vi "LoadMotorData.vi"(11 "Refnum in":T1) -> (3 "Refnum out":T1)   [LabVIEW 2014]
uses:
  <vilib>/Utility/config.llb/Config Data RefNum.ctl
  Variables/Physical data.vi
  <vilib>/Utility/config.llb/Read Key (Double).vi
  <vilib>/Utility/config.llb/Write Key (Double).vi
  <vilib>/Utility/config.llb/NI_LVConfig.lvlib
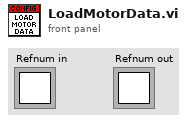
[diagram p1: front panel]
types:
  T1 = typedef "NI_LVConfig.lvlib/Config Data RefNum.ctl" = refnum<k1>
  T2 = cluster{"Free Current":dbl, "Stall Current":dbl, "Stall Torque":dbl, "Free Speed":dbl, "Gear Ratio":dbl, "Efficiency":dbl, "Moment":dbl}
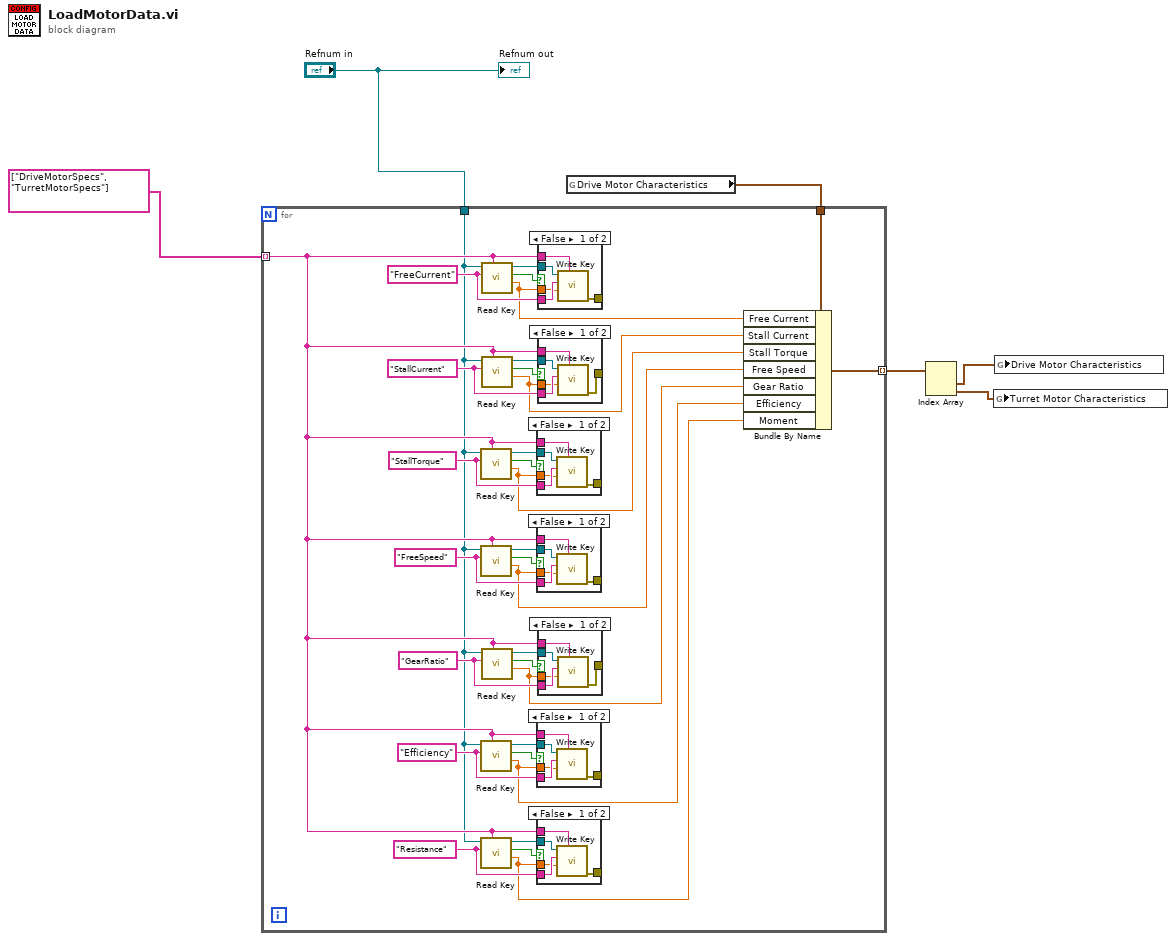
[diagram p0: block diagram]
diagram:
  n1 = global read "Physical data.vi" "Drive Motor Characteristics"() -> (w3:T2)
  n2 = for {
    tunnel: "Refnum in" -> [w16]
    tunnel: string[] ["DriveMotorSpecs", "TurretMotorSpecs"] -> [w17] mode=indexing
    tunnel: w3 -> [w15]
    tunnel: [w7] -> w4 mode=indexing
    w24 = "Resistance" ("string")
    w20 = "Efficiency" ("string")
    w23 = "GearRatio" ("string")
    w29 = "FreeSpeed" ("string")
    w33 = "StallTorque" ("string")
    w30 = "StallCurrent" ("string")
    w38 = "FreeCurrent" ("string")
    n3 = call-poly <vilib>:"Read Key.vi"("section"=w17, "key"=w33, "refnum"=w16) -> ("value"=w12:dbl, "found?"=w35:bool, "refnum out"=w34:T1)  [unwired: 5 in, 1 out]
    n4 = call-poly <vilib>:"Read Key.vi"("section"=w17, "key"=w29, "refnum"=w16) -> ("value"=w11:dbl, "found?"=w27:bool, "refnum out"=w28:T1)  [unwired: 5 in, 1 out]
    n5 = call-poly <vilib>:"Read Key.vi"("section"=w17, "key"=w20, "refnum"=w16) -> ("value"=w9:dbl, "found?"=w18:bool, "refnum out"=w19:T1)  [unwired: 5 in, 1 out]
    n6 = call-poly <vilib>:"Read Key.vi"("section"=w17, "key"=w24, "refnum"=w16) -> ("value"=w8:dbl, "found?"=w26:bool, "refnum out"=w25:T1)  [unwired: 5 in, 1 out]
    n7 = call-poly <vilib>:"Read Key.vi"("section"=w17, "key"=w38, "refnum"=w16) -> ("value"=w14:dbl, "found?"=w36:bool, "refnum out"=w37:T1)  [unwired: 5 in, 1 out]
    n8 = call-poly <vilib>:"Read Key.vi"("section"=w17, "key"=w30, "refnum"=w16) -> ("value"=w13:dbl, "found?"=w32:bool, "refnum out"=w31:T1)  [unwired: 5 in, 1 out]
    n9 = call-poly <vilib>:"Read Key.vi"("section"=w17, "key"=w23, "refnum"=w16) -> ("value"=w10:dbl, "found?"=w21:bool, "refnum out"=w22:T1)  [unwired: 5 in, 1 out]
    n10 = case shown="False" w35 {
      tunnel: w34 -> [w63 _]
      tunnel: w33 -> [w62 _]
      tunnel: w12 -> [w61 _]
      tunnel: w17 -> [w60 _]
      tunnel: [w59 _] -> _
      frame False {
        n11 = call-poly <vilib>:"Write Key.vi"("section"=w60, "value"=w61, "key"=w62, "refnum"=w63) -> ("error out"=w59:errorcluster)  [unwired: 5 in, 2 out]
      }
      frame True {
      }
    }
    n12 = case shown="False" w27 {
      tunnel: w28 -> [w58 _]
      tunnel: w29 -> [w57 _]
      tunnel: w11 -> [w56 _]
      tunnel: w17 -> [w55 _]
      tunnel: [w54 _] -> _
      frame False {
        n13 = call-poly <vilib>:"Write Key.vi"("section"=w55, "value"=w56, "key"=w57, "refnum"=w58) -> ("error out"=w54:errorcluster)  [unwired: 5 in, 2 out]
      }
      frame True {
      }
    }
    n14 = case shown="False" w18 {
      tunnel: w19 -> [w48 _]
      tunnel: w20 -> [w47 _]
      tunnel: w9 -> [w46 _]
      tunnel: w17 -> [w45 _]
      tunnel: [w44 _] -> _
      frame False {
        n15 = call-poly <vilib>:"Write Key.vi"("section"=w45, "value"=w46, "key"=w47, "refnum"=w48) -> ("error out"=w44:errorcluster)  [unwired: 5 in, 2 out]
      }
      frame True {
      }
    }
    n16 = case shown="False" w26 {
      tunnel: w25 -> [w43 _]
      tunnel: w24 -> [w42 _]
      tunnel: w8 -> [w41 _]
      tunnel: w17 -> [w40 _]
      tunnel: [w39 _] -> _
      frame False {
        n17 = call-poly <vilib>:"Write Key.vi"("section"=w40, "value"=w41, "key"=w42, "refnum"=w43) -> ("error out"=w39:errorcluster)  [unwired: 5 in, 2 out]
      }
      frame True {
      }
    }
    n18 = case shown="False" w36 {
      tunnel: w37 -> [w73 _]
      tunnel: w38 -> [w72 _]
      tunnel: w14 -> [w71 _]
      tunnel: w17 -> [w70 _]
      tunnel: [w69 _] -> _
      frame False {
        n19 = call-poly <vilib>:"Write Key.vi"("section"=w70, "value"=w71, "key"=w72, "refnum"=w73) -> ("error out"=w69:errorcluster)  [unwired: 5 in, 2 out]
      }
      frame True {
      }
    }
    n20 = case shown="False" w32 {
      tunnel: w31 -> [w68 _]
      tunnel: w30 -> [w67 _]
      tunnel: w13 -> [w66 _]
      tunnel: w17 -> [w65 _]
      tunnel: [w64 _] -> _
      frame False {
        n21 = call-poly <vilib>:"Write Key.vi"("section"=w65, "value"=w66, "key"=w67, "refnum"=w68) -> ("error out"=w64:errorcluster)  [unwired: 5 in, 2 out]
      }
      frame True {
      }
    }
    n22 = case shown="False" w21 {
      tunnel: w22 -> [w53 _]
      tunnel: w23 -> [w52 _]
      tunnel: w10 -> [w51 _]
      tunnel: w17 -> [w50 _]
      tunnel: [w49 _] -> _
      frame False {
        n23 = call-poly <vilib>:"Write Key.vi"("section"=w50, "value"=w51, "key"=w52, "refnum"=w53) -> ("error out"=w49:errorcluster)  [unwired: 5 in, 2 out]
      }
      frame True {
      }
    }
    n24 = Bundle By Name(cluster=w15, "Free Current"=w14, "Stall Current"=w13, "Stall Torque"=w12, "Free Speed"=w11, "Gear Ratio"=w10, "Efficiency"=w9, "Moment"=w8) -> (w7:T2)
  }
  n25 = Index Array(array=w4) -> (element #1=w5:T2, element #2=w6:T2)  [unwired: 2 in]
  n26 = global write "Physical data.vi" "Turret Motor Characteristics"(w6) -> ()
  n27 = global write "Physical data.vi" "Drive Motor Characteristics"(w5) -> ()
  "Refnum out" <- "Refnum in"
